vi "NXT_MIDBRAIN_BEHAVIOR Master Brain.vi"(4 "_fromPC":u8[](array[numeric]), 5 "_behaviorWeights":T3) -> (0 "_irTheta":i8, 1 "_behaviorData":T2[](array[typedef]))   [LabVIEW 2012, in "Tugboat.lvrbt"]
uses:
  Tugboat.lvrbt
  behaviorWeights_t.ctl
  behaviorOutput_t.ctl
  motorCommands_t.ctl
panel:
  in  "_motorCommands":T1={"_rudderCommand"=7, "_propCommand"=7, "_irServoCommand"=7}
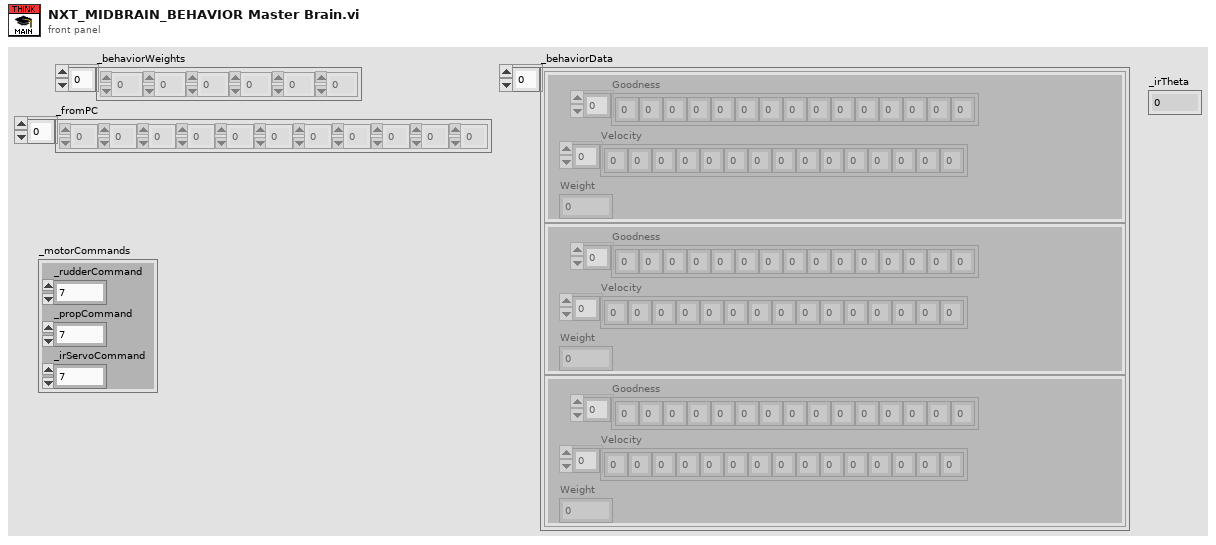
[diagram p1: front panel]
types:
  T1 = typedef "motorCommands_t.ctl" = cluster{"_rudderCommand":i8, "_propCommand":i8, "_irServoCommand":i8}
  T2 = typedef "behaviorOutput_t.ctl" = cluster{"Goodness":i8[], "Velocity":i8[], "Weight":i8}
  T3 = typedef "behaviorWeights_t.ctl" = i8[]
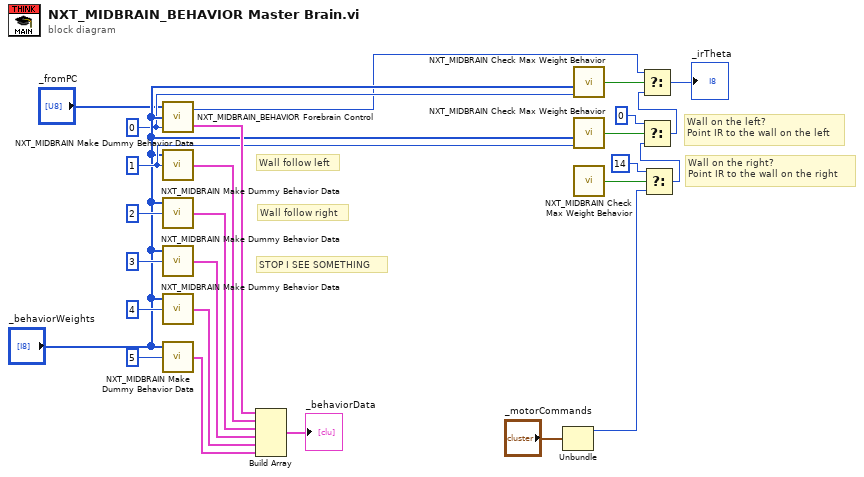
[diagram p0: block diagram]
diagram:
  w12 = 0 ("Behavior #")
  w15 = 1 ("Behavior #")
  # "Wall on the right? \nPoint IR to the wall on the right"
  # "Wall on the left? \nPoint IR to the wall on the left"
  # "STOP I SEE SOMETHING"
  # "Wall follow right"
  # "Wall follow left"
  n1 = call "NXT_MIDBRAIN_BEHAVIOR Forebrain Control.vi"("Behavior #"=w12, "_behaviorWeights"="_behaviorWeights", "_fromPC"="_fromPC") -> ("_behaviorOutput"=w22:T2, "_FBirTheta"=w8:i8)
  n2 = call "NXT_MIDBRAIN Make Dummy Behavior Data.vi"("Behavior #"=w15, "Behavior Weights"="_behaviorWeights") -> ("Behavior Output"=w21:T2)  [unwired: 1 in]
  n3 = call "NXT_MIDBRAIN Make Dummy Behavior Data.vi"("Behavior #"=2, "Behavior Weights"="_behaviorWeights") -> ("Behavior Output"=w20:T2)  [unwired: 1 in]
  n4 = call "NXT_MIDBRAIN Make Dummy Behavior Data.vi"("Behavior #"=3, "Behavior Weights"="_behaviorWeights") -> ("Behavior Output"=w19:T2)  [unwired: 1 in]
  n5 = call "NXT_MIDBRAIN Make Dummy Behavior Data.vi"("Behavior #"=4, "Behavior Weights"="_behaviorWeights") -> ("Behavior Output"=w18:T2)  [unwired: 1 in]
  n6 = call "NXT_MIDBRAIN Make Dummy Behavior Data.vi"("Behavior #"=5, "Behavior Weights"="_behaviorWeights") -> ("Behavior Output"=w17:T2)  [unwired: 1 in]
  n7 = Build Array(w22, w21, w20, w19, w18, w17) -> (→"_behaviorData":T2[])
  n8 = Unbundle("_motorCommands") -> ("_rudderCommand"=w2:i8)  [unwired: 2 out]
  n9 = call "NXT_MIDBRAIN Check Max Weight Behavior.vi"("Behavior #"=w12, "_behaviorWeights"="_behaviorWeights") -> ("Max?"=w9:bool)  [unwired: 2 in]
  n10 = call "NXT_MIDBRAIN Check Max Weight Behavior.vi"("Behavior #"=w15, "_behaviorWeights"="_behaviorWeights") -> ("Max?"=w14:bool)  [unwired: 2 in]
  n11 = call "NXT_MIDBRAIN Check Max Weight Behavior.vi"() -> ("Max?"=w3:bool)  [unwired: 4 in]
  n12 = Select(t=i8 14, s=w3, f=w2) -> (s? t:f=w1:i8)
  n13 = Select(t=i8 0, s=w14, f=w1) -> (s? t:f=w6:i8)
  n14 = Select(t=w8, s=w9, f=w6) -> (s? t:f=→"_irTheta":i8)
